vi "LJM logger filter inf values.vi"(1 "InValues":dbl[](array[numeric])=[0.0, 0.0]) -> (0 "OutValues":dbl[](array[numeric]))   [LabVIEW 2026]
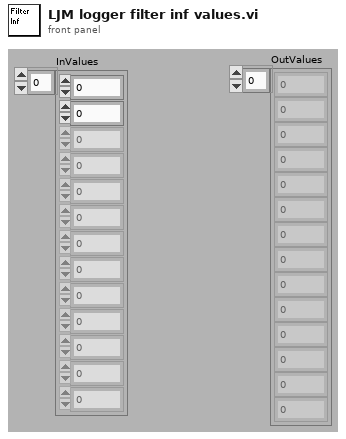
[diagram p1: front panel]
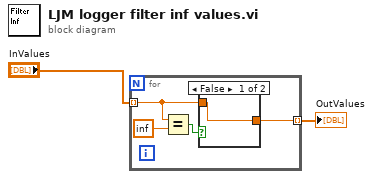
[diagram p0: block diagram]
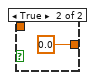
[diagram p2: hidden frame]
diagram:
  n1 = for {
    tunnel: "InValues" -> [w5] mode=indexing
    tunnel: [w4] -> w1 mode=indexing
    n2 = Equal?(x=w5, y=inf) -> (x = y?=w6:bool)
    n3 = case shown="False" w6 {
      tunnel: [w7 0.0] -> w4
      tunnel: w5 -> [w7 _]
      frame False {
      }
      frame True {
      }
    }
  }
  "OutValues" <- w1
